vi "Covtype.vi"(8 "error in (no error)":errorcluster caption="entrée d'erreur (pas d'erreur)", 11 "fetch_covtype":T2={"download_if_missing"=TRUE, "random_state"=-1, "shuffle"=TRUE, "Returns"="Data"} {"random_state" min=-1}) -> (0 "error out":errorcluster, 3 "Data":T1)   [LabVIEW 2020]
doc: "The samples in this dataset correspond to 30×30m patches of forest in the US, collected for the task of predicting each patch’s cover type, i.e. the dominant species of tree. There are seven covertypes, making this a multiclass classification problem. Each sample has 54 features, described on the dataset’s homepage. Some of the features are boolean indicators, while others are discrete or continuous measurements.\n\nData Set Characteristics :\n - Classes : 7\n - Samples total : 581012\n - Dimensionality : 54\n - Features : int\n\nParameters :\n\n- download_if_missing : boolean, default=True\nIf False, raise a IOError if the data is not locally available instead of trying to download the data from the source site.\n\n- random_state : int, RandomState instance, default=None=-1\nDetermines random number generation for dataset shuffling. Pass an int for reproducible output across multiple function calls. See Glossary.\n\n- shuffle : bool, default=False\nWhether to shuffle dataset.\n\nReturns :\n\n- data : numpy array of shape (581012, 54)\nEach row corresponds to the 54 features in the dataset.\n\n- target : numpy array of shape (581012,)\nEach value corresponds to one of the 7 forest covertypes with values ranging between 1 to 7."
uses:
  Covtype.lvclass
panel:
  out "Covtype.lvclass":refnum<class "Covtype.lvclass">
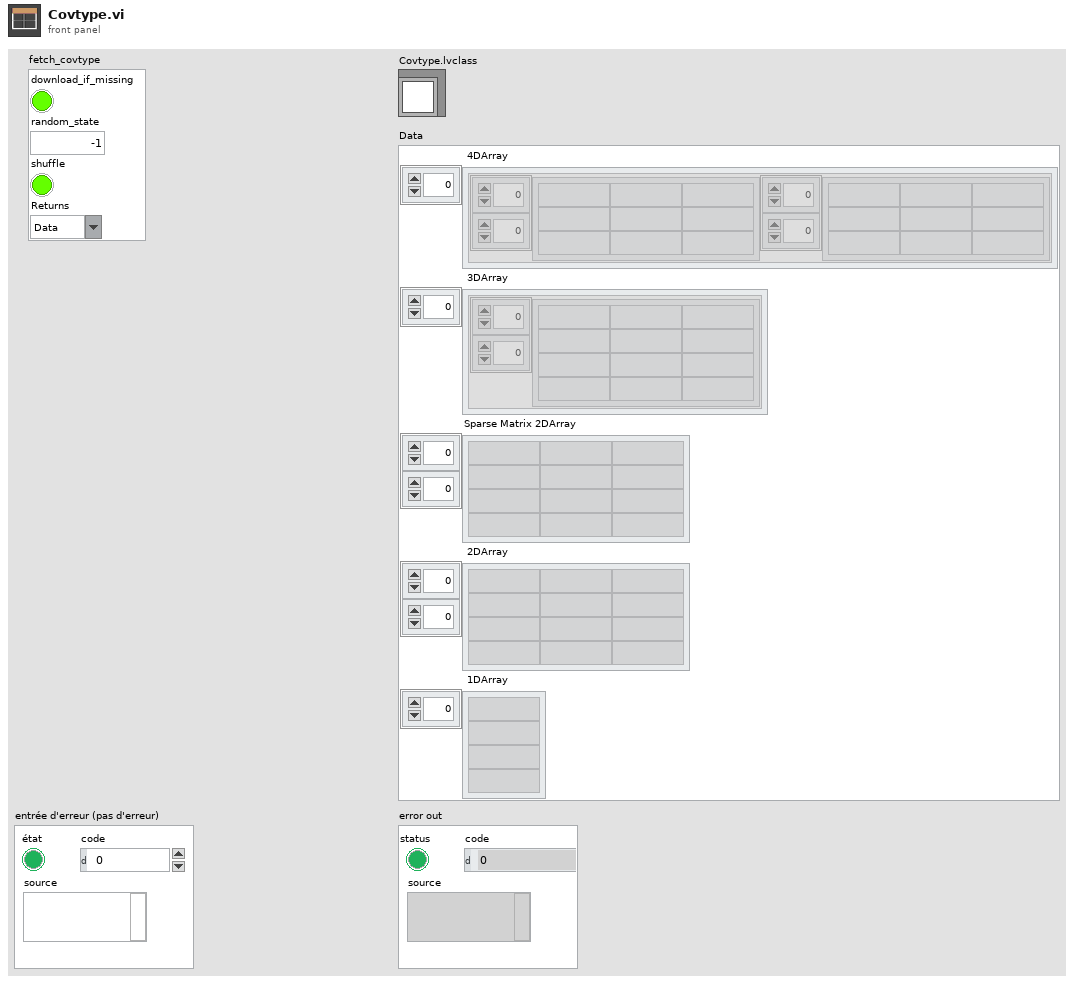
[diagram p1: front panel]
types:
  T1 = cluster{" 4DArray":cluster{"1":string[][], "2":string[][]}[], " 3DArray":cluster{"Tableau":string[][]}[], "Sparse Matrix 2DArray":string[][], " 2DArray":string[][], " 1DArray":string[]}
  T2 = cluster{"download_if_missing":bool, "random_state":i32, "shuffle":bool, "Returns":string}
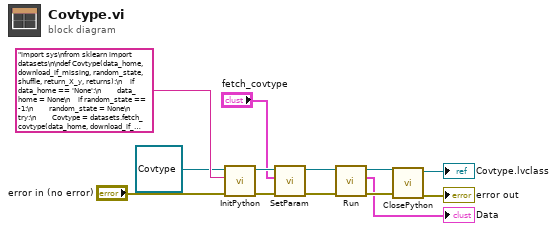
[diagram p0: block diagram]
diagram:
  n1 = call-dynamic "InitPython.vi"("error in (no error)"="error in (no error)", "Python Instruction"="import sys\nfrom sklearn import datasets\n\ndef Covtype(data_home, download_if_missing, random_state, shuffle, return_X_y, returns):\n    if data_home == 'None':\n        data_home = None\n    if random_state == -1:\n        random_state = None\n    try:\n        Covtype = datasets.fetch_covtype(data_home, download_if_missing, random_state, shuffle, return_X_y)\n        if returns == 'Data' : \n            data = Covtype['data'].tolist()\n            return str(data)\n        else :\n            data = Covtype['target'].tolist()\n            return str(data)\n    except:\n        erreur = sys.exc_info()\n        typerr = u\"%s\" % (erreur[0])\n        typerr = typerr[typerr.find(\"'\")+1:typerr.rfind(\"'\")]\n        msgerr = u\"%s\" % (erreur[1])\n        message = str('/!\\\\ {0} : {1}'. format(typerr,msgerr))\n        return message", "Scikit-learn en entrée"=refnum<class "Covtype.lvclass"> refnum ("Covtype.lvclass")) -> ("error out"=w10:errorcluster, "Scikit-learn en sortie"=w11:refnum<class "Covtype.lvclass">)  [unwired: 7 in]
  n2 = call-dynamic "SetParam.vi"("error in (no error)"=w10, "fetch_covtype"="fetch_covtype", "Covtype.lvclass"=w11) -> ("error out"=w6:errorcluster, "Covtype.lvclass"=w7:refnum<class "Covtype.lvclass">)  [unwired: 7 in]
  n3 = call-dynamic "Run.vi"("error in (no error)"=w6, "Covtype.lvclass"=w7) -> ("error out"=w4:errorcluster, "Data"=→"Data":T1, "Covtype.lvclass"=w5:refnum<class "Covtype.lvclass">)  [unwired: 7 in]
  n4 = call-dynamic "ClosePython.vi"("error in (no error)"=w4, "Scikit-learn en entrée"=w5) -> ("error out"=→"error out":errorcluster, "Scikit-learn en sortie"=→"Covtype.lvclass":refnum<class "Covtype.lvclass">)  [unwired: 8 in]
